vi "Get All.vi"(11 "Entity Collection in":refnum<class "Entity Collection.lvclass">) -> (2 "Entities":refnum<class "Entity.lvclass">[](array[class]))   [LabVIEW 2020, in "Conditu2.lvlib" / "Columns.lvlib" / "Entity Collection.lvclass"]
uses:
  Entity Collection.lvclass
  Entity/Entity.lvclass
  Entity Collection.lvclass/Entity Collection.ctl
  c7fb9928-d132-4eb5-82f4-915fb747de2a.vi
  <vilib>/Comparison/Less/Less Functor/Less Functor.lvclass
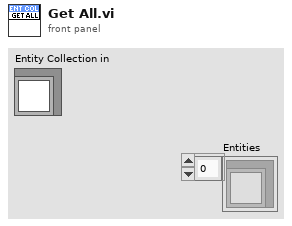
[diagram p1: front panel]
types:
  T1 = typedef "Conditu2.lvlib/Entity ID.ctl" = i64
  T2 = typedef "Conditu2.lvlib/Columns.lvlib/Entity Collection.lvclass/Entity Sort.ctl" = cluster{"Order":u64, "Entity":refnum<class "Entity.lvclass">}
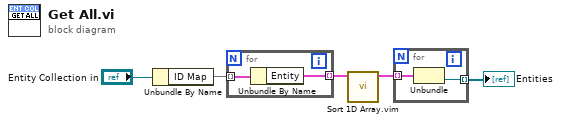
[diagram p0: block diagram]
diagram:
  n1 = Unbundle By Name("Entity Collection in") -> ("ID Map"=w4:map{T1, T2})
  n2 = for {
    tunnel: w4 -> [w7] mode=indexing
    tunnel: [w6] -> w3 mode=indexing
    n3 = Unbundle By Name(w7) -> ("Entity"=w6:T2)
  }
  n4 = call "Sort 1D Array.vim"("unsorted array"=w3) -> ("sorted array"=w2:T2[])  [unwired: 10 in]
  n5 = for {
    tunnel: w2 -> [w9] mode=indexing
    tunnel: [w8] -> w1 mode=indexing
    n6 = Unbundle(w9) -> ("Entity"=w8:refnum<class "Entity.lvclass">)  [unwired: 1 out]
  }
  "Entities" <- w1
